vi "NormalizeLUT.vi"(11 "LUT":sgl[][](array[numeric])) -> (3 "Array":sgl[][](array[numeric]))   [LabVIEW 2011]
panel:
  out "Normalize LUT":sgl[][](graph)
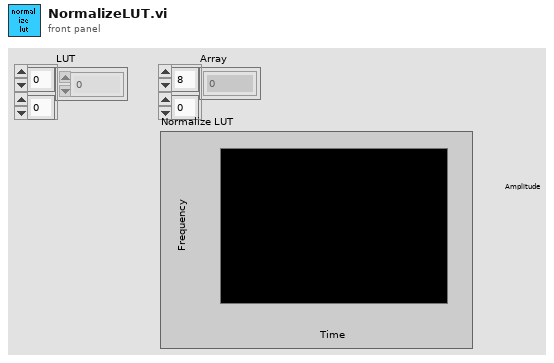
[diagram p1: front panel]
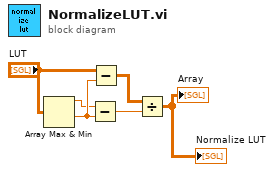
[diagram p0: block diagram]
diagram:
  n1 = Array Max & Min(array="LUT") -> (max value=w4:sgl, min value=w5:sgl)  [unwired: 2 out]
  n2 = Subtract(x=w4, y=w5) -> (x-y=w6:sgl)
  n3 = Subtract(x="LUT", y=w5) -> (x-y=w3:sgl[][])
  n4 = Divide(x=w3, y=w6) -> (x/y=→"Array" →"Normalize LUT":sgl[][])
